vi "read configuration.vi"() -> (0 "Waveform Generator IO":string, 2 "Oscilloscope IO":string)   [LabVIEW 2016]
uses:
  <vilib>/Utility/config.llb/Read Key (String).vi
  <vilib>/Utility/config.llb/NI_LVConfig.lvlib
panel:
  out "连接的字符串":string
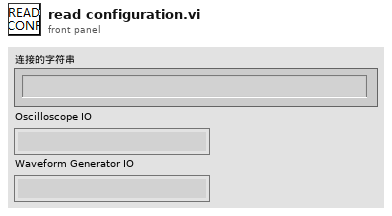
[diagram p1: front panel]
types:
  T1 = typedef "NI_LVConfig.lvlib/Config Data RefNum.ctl" = refnum<k1>
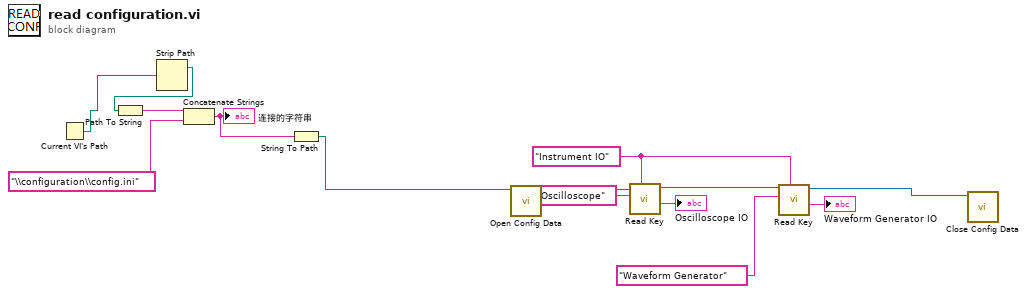
[diagram p0: block diagram]
diagram:
  w5 = "Instrument IO" ("section")
  n1 = Current VI's Path() -> (path=w13:path)
  n2 = Strip Path(path=w13) -> (stripped path=w12:path)  [unwired: 1 out]
  n3 = Path To String(path=w12) -> (string=w11:string)
  n4 = Concatenate Strings(w11, "\\configuration\\config.ini" ("字符串")) -> (w10:string)
  "连接的字符串" <- w10
  n5 = String To Path(string=w10) -> (path=w9:path)
  n6 = call <vilib>:"Open Config Data.vi"("configuration file path"=w9) -> ("refnum"=w8:T1)  [unwired: 8 in, 2 out]
  n7 = call-poly <vilib>:"Read Key.vi"("section"=w5, "key"="Oscilloscope", "refnum"=w8) -> ("value"=→"Oscilloscope IO":string, "refnum out"=w4:T1)  [unwired: 5 in, 2 out]
  n8 = call-poly <vilib>:"Read Key.vi"("section"=w5, "key"="Waveform Generator", "refnum"=w4) -> ("value"=→"Waveform Generator IO":string, "refnum out"=w1:T1)  [unwired: 5 in, 2 out]
  n9 = call <vilib>:"Close Config Data.vi"("refnum"=w1) -> ()  [unwired: 9 in, 2 out]
